vi "Generate Event.vi"(8 "error in (no error)":errorcluster caption="entrée d'erreur (pas d'erreur)", 9 "Data":variant, 10 "Command":T1, 11 "Message en entrée":refnum<class "Message.lvclass">) -> (0 "error out":errorcluster caption="sortie d'erreur", 3 "Message en sortie":refnum<class "Message.lvclass">)   [LabVIEW 2018, in "Message.lvclass"]
uses:
  Message.lvclass
  dependecies/ControlsVIs/Clusters-def/SERVER-Commands.ctl
  Message.lvclass/Message.ctl
  Control/Control-Server/Control-Server.lvclass
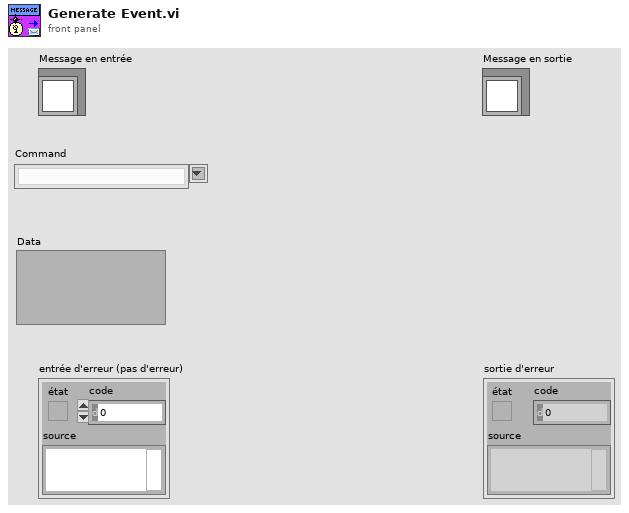
[diagram p1: front panel]
types:
  T1 = typedef "Control-Server.lvclass/SERVER-Commands.ctl" = string
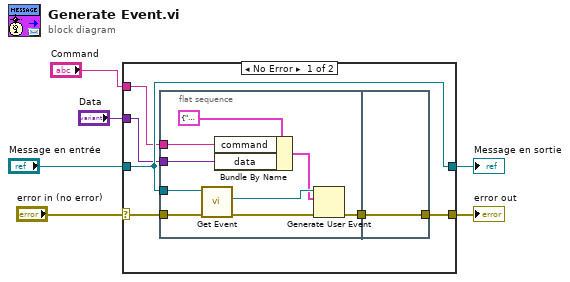
[diagram p0: block diagram]
diagram:
  n1 = case shown="No Error" "error in (no error)" {
    selector: "error in (no error)" -> [w11 w24]
    tunnel: [w10 w24] -> w5
    tunnel: [w12 w23] -> w3
    tunnel: "Message en entrée" -> [w12 w23]
    tunnel: "Command" -> [w9 _]
    tunnel: "Data" -> [w8 _]
    frame No Error {
      n2 = flat-sequence {
        tunnel: w12 -> [w21]
        tunnel: w11 -> [w19]
        tunnel: w9 -> [w15]
        tunnel: w8 -> [w14]
        tunnel: [w17] -> w7
        tunnel: [w22] -> w10
        tunnel: w7 -> [w22]
        frame #0 {
          n3 = call "Get Event.vi"("error in (no error)"=w19, "Message en entrée"=w21) -> ("error out"=w18:errorcluster, "UserEventCommand"=w20:refnum<user-event>)  [unwired: 7 in, 1 out]
          n4 = Bundle By Name(cluster=cluster{"command":string, "data":variant} {"command"="", "data"=variant} ("données d'événement"), "command"=w15, "data"=w14) -> (w13:cluster{"command":string, "data":variant})
          n5 = Generate User Event(user event=w20, event data cluster=w13, error in=w18) -> (error out=w17:errorcluster)  [unwired: 1 in, 1 out]
        }
        frame #1 {
        }
      }
    }
    frame Error {
    }
  }
  "error out" <- w5
  "Message en sortie" <- w3
